vi "Get Node.vi"(8 "error in (no error)":errorcluster, 10 "Node":string, 11 "Test Result in":refnum<class "Test Result.lvclass">) -> (0 "error out":errorcluster, 1 "Assertions":T3[](array[typedef]), 2 "Test Node":T1, 3 "Test Result out":refnum<class "Test Result.lvclass">, 4 "found":bool, 5 "indent level":i32)   [LabVIEW 2013, in "Caraya.lvlib" / "Test Result.lvclass"]
uses:
  Test Result.lvclass
  Assert Event Data.ctl
  Test Node.ctl
  Test Registration Data.ctl
  Test Result.lvclass/Test Result.ctl
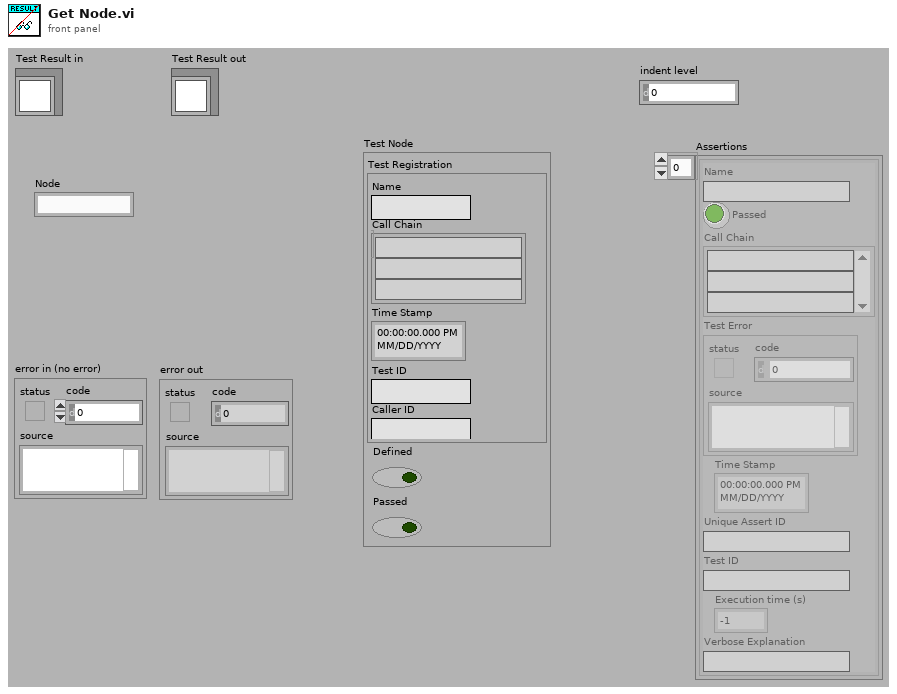
[diagram p1: front panel]
types:
  T1 = typedef "Caraya.lvlib/Test Result.lvclass/Test Node.ctl" = cluster{"Test Registration":T2, "Defined":bool, "Passed":bool}
  T2 = typedef "Caraya.lvlib/Test Result.lvclass/Test Registration Data.ctl" = cluster{"Name":string, "Call Chain":string[], "Time Stamp":timestamp, "Test ID":string, "Caller ID":string}
  T3 = typedef "Caraya.lvlib/Test Result.lvclass/Assert Event Data.ctl" = cluster{"Name":string, "Passed":bool, "Call Chain":string[], "Test Error":errorcluster, "Time Stamp":timestamp, "Unique Assert ID":string, "Test ID":string, "Execution time (s)":dbl, "Verbose Explanation":string}
  T4 = typedef "Caraya.lvlib/Test Result.lvclass/Node Results (Extended).ctl" = cluster{"Test Node":T5, "Assertions":T6[]}
  T5 = typedef "Caraya.lvlib/Test Result.lvclass/Test Node (Extended).ctl" = cluster{"Test Registration":T2, "Defined":bool, "Passed":bool, "properties":variant}
  T6 = typedef "Caraya.lvlib/Test Result.lvclass/Assert Event Data (Extended).ctl" = cluster{"Name":string, "Passed":bool, "Call Chain":string[], "Test Error":errorcluster, "Time Stamp":timestamp, "Unique Assert ID":string, "Test ID":string, "Execution time (s)":dbl, "Verbose Explanation":string, "properties":variant, "measurements":variant, "limits":variant}
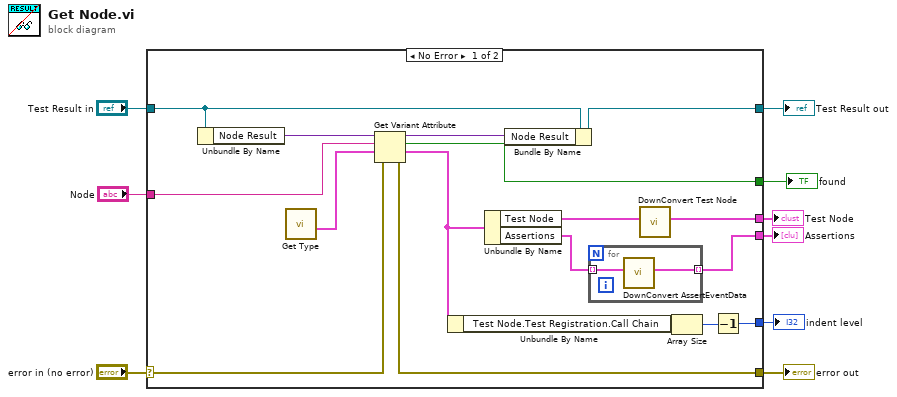
[diagram p0: block diagram]
diagram:
  n1 = case shown="No Error" "error in (no error)" {
    selector: "error in (no error)" -> [w21 w30]
    tunnel: [w22 w30] -> w8
    tunnel: [w25 w29] -> w6
    tunnel: "Test Result in" -> [w26 w29]
    tunnel: "Node" -> [w20 _]
    tunnel: [w19 _] -> w4
    tunnel: [w10 _] -> w2
    tunnel: [w12 _] -> w3
    tunnel: [w15 _] -> w1
    frame No Error {
      n2 = Unbundle By Name(w26) -> ("Node Result"=w24:variant)
      n3 = call "Get Type.vi"() -> ("Extended Node Result"=w14:T4)  [unwired: 10 in, 1 out]
      n4 = Get Variant Attribute(Variant=w24, name=w20, default value (empty Variant)=w14, error in=w21) -> (duplicate Variant=w23:variant, found=w19:bool, value=w18:T4, error out=w22:errorcluster)
      n5 = Unbundle By Name(w18) -> ("Test Node.Test Registration.Call Chain"=w17:string[])
      n6 = Unbundle By Name(w18) -> ("Test Node"=w11:T5, "Assertions"=w13:T6[])
      n7 = Bundle By Name(cluster=w26, "Node Result"=w23) -> (w25:refnum<class "Test Result.lvclass">)
      n8 = for {
        tunnel: w13 -> [w28] mode=indexing
        tunnel: [w27] -> w12 mode=indexing
        n9 = call "DownConvert AssertEventData.vi"("Assert Event Data (Extended)"=w28) -> ("Assert Event Data"=w27:T3)  [unwired: 10 in]
      }
      n10 = call "DownConvert Test Node.vi"("Test Node (Extended)"=w11) -> ("Test Node"=w10:T1)  [unwired: 10 in]
      n11 = Array Size(array=w17) -> (size(s)=w16:i32)
      n12 = Decrement(x=w16) -> (x-1=w15:i32)
    }
    frame Error {
    }
  }
  "error out" <- w8
  "Test Result out" <- w6
  "found" <- w4
  "Assertions" <- w3
  "Test Node" <- w2
  "indent level" <- w1
